vi "KE6221 -- Get Wave Type.vi"(0 "Resource In":refnum<visa-resource-name>, 1 "Check For SCPI Errors? (T)":bool=TRUE, 11 "error in (no error)":errorcluster) -> (4 "Resource Out (dupl)":refnum<visa-resource-name>, 8 "KE6221 Wave Type":T1=enum."Square", 15 "error out":errorcluster)   [LabVIEW 2019, in "Keithley 622x.lvlib"]
uses:
  Keithley 622x.lvlib
  Low Level/Typedefs/KE6221 -- Wave Type.ctl
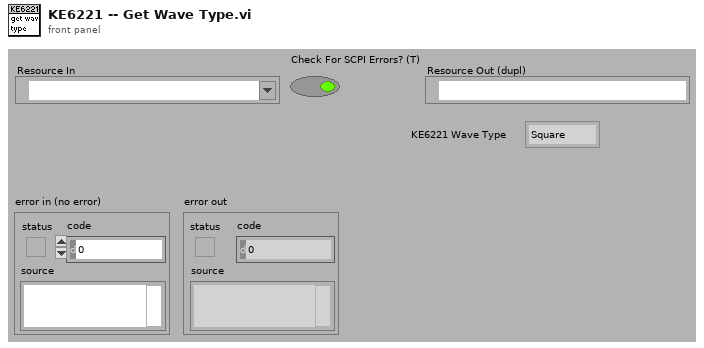
[diagram p1: front panel]
types:
  T1 = typedef "Keithley 622x.lvlib/KE6221 -- Wave Type.ctl" = enum16{"Sinusoid", "Square", "Ramp", "Arbitrary 0", "Arbitrary 1", "Arbitrary 2", "Arbitrary 3", "Arbitrary 4"}
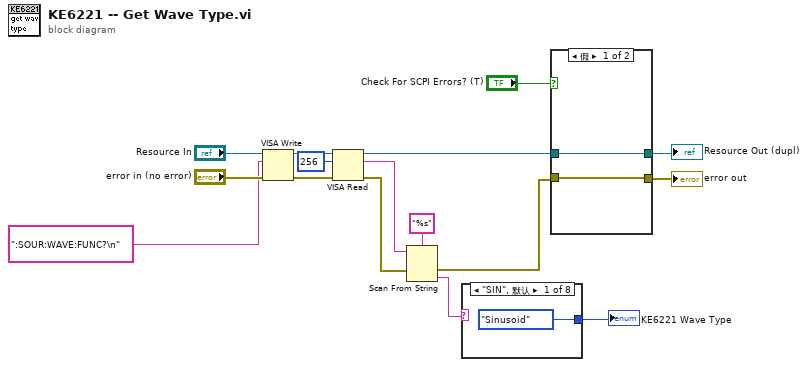
[diagram p0: block diagram]
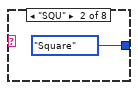
[diagram p2: hidden frame]
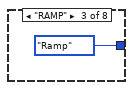
[diagram p3: hidden frame]
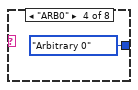
[diagram p4: hidden frame]
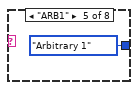
[diagram p5: hidden frame]
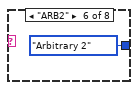
[diagram p6: hidden frame]
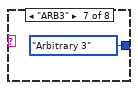
[diagram p7: hidden frame]
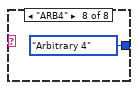
[diagram p8: hidden frame]
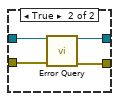
[diagram p9: hidden frame]
diagram:
  n1 = VISA Write(VISA resource name="Resource In", write buffer=":SOUR:WAVE:FUNC?\n" ("format string"), error in (no error)="error in (no error)") -> (VISA resource name out=w10:refnum<visa-resource-name>, error out=w9:errorcluster)  [unwired: 1 out]
  n2 = VISA Read(VISA resource name=w10, byte count=u32 256, error in (no error)=w9) -> (VISA resource name out=w3:refnum<visa-resource-name>, read buffer=w5:string, error out=w7:errorcluster)  [unwired: 1 out]
  n3 = Scan From String(format string="%s", input string=w5, error in=w7) -> (error out=w4:errorcluster, output 1=w2:string)  [unwired: 2 in, 2 out]
  n4 = case shown="\"SIN\", 默认" w2 {
    tunnel: [KE6221_--_Wave_Type."Sinusoid" ("KE6221 Wave Type") KE6221_--_Wave_Type."Square" ("KE6221 Wave Type") KE6221_--_Wave_Type."Ramp" ("KE6221 Wave Type") KE6221_--_Wave_Type."Arbitrary 0" ("KE6221 Wave Type") KE6221_--_Wave_Type."Arbitrary 1" ("KE6221 Wave Type") KE6221_--_Wave_Type."Arbitrary 2" ("KE6221 Wave Type") KE6221_--_Wave_Type."Arbitrary 3" ("KE6221 Wave Type") KE6221_--_Wave_Type."Arbitrary 4" ("KE6221 Wave Type")] -> w1
    frame "SIN", Default {
    }
    frame "SQU" {
    }
    frame "RAMP" {
    }
    frame "ARB0" {
    }
    frame "ARB1" {
    }
    frame "ARB2" {
    }
    frame "ARB3" {
    }
    frame "ARB4" {
    }
  }
  "KE6221 Wave Type" <- w1
  n5 = case shown="假" "Check For SCPI Errors? (T)" {
    tunnel: w3 -> [w26 w30]
    tunnel: w4 -> [w25 w29]
    tunnel: [w25 w28] -> w12
    tunnel: [w26 w27] -> w13
    frame False {
    }
    frame True {
      n6 = call "Error Query.vi"("VISA Resource In"=w30, "error in (no error)"=w29) -> ("VISA Resource Out (dupl)"=w27:refnum<visa-resource-name>, "error out"=w28:errorcluster)  [unwired: 10 in, 2 out]
    }
  }
  "Resource Out (dupl)" <- w13
  "error out" <- w12
